vi "Publish Services.vi"(8 "error in (no error)":errorcluster, 11 "CS++DIM-Server in":refnum<class "CS++DIM-Server.lvclass">) -> (0 "error out":errorcluster, 3 "CS++DIM-Server out":refnum<class "CS++DIM-Server.lvclass">)   [LabVIEW 2014, in "CS++DIM-Server.lvlib" / "CS++DIM-Server.lvclass"]
doc: "Publish PV."
uses:
  CS++DIM-Server.lvclass
  CSPP_Core/Actors/CS++BaseActor/CS++BaseActor.lvclass/CS++BaseActor.ctl
  CS++DIM-Server.lvclass/CS++DIM-Server.ctl
  CSPP_Core/Classes/CS++ProcessVariables/PVConnection/PVConnection.lvclass/PVConnection.ctl
  CSPP_Core/Classes/CS++ProcessVariables/ProcessVariable/PV.lvclass/PV.ctl
  <vilib>/ActorFramework/Actor/Actor.lvclass/Actor.ctl
  <vilib>/ActorFramework/Message Enqueuer/Message Enqueuer.lvclass/Message Enqueuer.ctl
  <vilib>/ActorFramework/Message Enqueuer/Init from Existing Queue.vi
  <vilib>/ActorFramework/Message Enqueuer/Enqueue.vi
  <vilib>/ActorFramework/Message Priority Queue/Priority Enqueue.vi
  CSPP_Core/Classes/CS++ProcessVariables/ProcessVariable/PV.lvclass
  <vilib>/ActorFramework/Message Enqueuer/Message Enqueuer.lvclass
  CS++DIM-Server Messages/Publish Services Msg/Publish Services Msg.lvclass
  CSPP_Core/Actors/CS++BaseActor/CS++BaseActor.lvclass
  CSPP_Core/Classes/CS++ProcessVariables/PVConnection/PVConnection.lvclass
  <vilib>/ActorFramework/Actor/Actor.lvclass
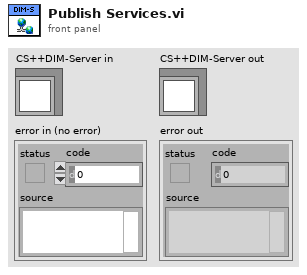
[diagram p1: front panel]
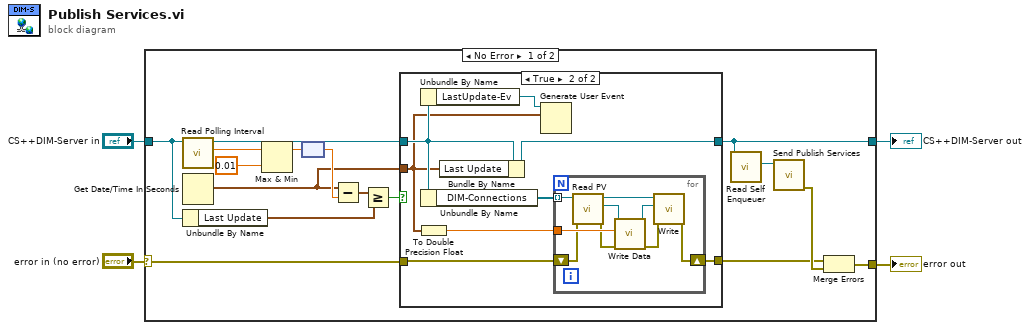
[diagram p0: block diagram]
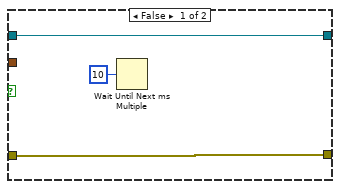
[diagram p2: hidden frame]
diagram:
  n1 = case shown="No Error" "error in (no error)" {
    selector: "error in (no error)" -> [w10 w42]
    tunnel: [w6 w42] -> w3
    tunnel: [w9 w41] -> w1
    tunnel: "CS++DIM-Server in" -> [w19 w41]
    frame No Error {
      n2 = call "Read Polling Interval.vi"("CS++BaseActor in"=w19) -> ("Polling Interval"=w16:dbl[unit], "CS++BaseActor out"=w12:refnum<class "CS++DIM-Server.lvclass">)  [unwired: 8 in, 1 out]
      n3 = Get Date/Time In Seconds() -> (seconds since 1Jan1904=w11:timestamp)
      n4 = Unbundle By Name(w19) -> ("Last Update"=w17:timestamp)
      n5 = Max & Min(x=w16, y=dbl[unit] 0.01) -> (max(x,y)=w15:dbl[unit])  [unwired: 1 out]
      n6 = node(w15) -> (w20:dbl)
      n7 = Subtract(x=w11, y=w20) -> (x-y=w18:timestamp)
      n8 = Greater Or Equal?(x=w18, y=w17) -> (x >= y?=w13:bool)
      n9 = case shown="True" w13 {
        tunnel: w12 -> [w23 w26]
        tunnel: w11 -> [_ w24]
        tunnel: [w23 w31] -> w9
        tunnel: w10 -> [w21 w28]
        tunnel: [w21 w29] -> w5
        frame False {
          n10 = Wait Until Next ms Multiple(millisecond multiple=u32 10) -> ()  [unwired: 1 out]
        }
        frame True {
          n11 = To Double Precision Float(number=w24) -> (double precision float=w27:dbl)
          n12 = Unbundle By Name(w26) -> ("LastUpdate-Ev"=w25:refnum<user-event>)
          n13 = Unbundle By Name(w26) -> ("DIM-Connections"=w30:refnum<class "PVConnection.lvclass">[])
          n14 = Bundle By Name(cluster=w26, "Last Update"=w24) -> (w31:refnum<class "CS++DIM-Server.lvclass">)
          n15 = Generate User Event(user event=w25, event data cluster=w24) -> ()  [unwired: 2 in, 2 out]
          n16 = for {
            tunnel: w30 -> [w39] mode=indexing
            shift-right: [w40] -> w29
            shift-left: w28 -> [w33]
            tunnel: w27 -> [w35]
            n17 = call "Read PV.vi"("error in (no error)"=w33, "PVConnection in"=w39) -> ("error out"=w34:errorcluster, "PV"=w36:refnum<class "PV.lvclass">, "PVConnection out"=w38:refnum<class "PVConnection.lvclass">)  [unwired: 7 in]
            n18 = call "Write Data.vi"("error in (no error)"=w34, "Data"=w35, "PV in"=w36) -> ("error out"=w32:errorcluster, "PV out"=w37:refnum<class "PV.lvclass">)  [unwired: 7 in]
            n19 = call "Write.vi"("error in (no error)"=w32, "PV"=w37, "PVConnection in"=w38) -> ("error out"=w40:errorcluster)  [unwired: 7 in, 1 out]
          }
        }
      }
      n20 = call <vilib>:"Read Self Enqueuer.vi"("Actor"=w9) -> ("Self Enqueuer"=w8:refnum<class "Message Enqueuer.lvclass">)  [unwired: 10 in]
      n21 = call "Send Publish Services.vi"("Message Enqueuer"=w8) -> ("error out"=w7:errorcluster)  [unwired: 9 in, 1 out]
      n22 = Merge Errors(w5, w7) -> (w6:errorcluster)
    }
    frame Error {
    }
  }
  "error out" <- w3
  "CS++DIM-Server out" <- w1
